vi "Fpga-ItchParser-TestHarness.vi"   [LabVIEW 2016]
uses:
  <vilib>/Platform/TimedLoop/XDataNode/timing_clust.ctl
  <vilib>/Platform/TimedLoop/XDataNode/nitl_modes.ctl
  <vilib>/Platform/TimedLoop/XDataNode/wakeup.ctl
  <vilib>/rvi/Emulation/niFpgaSctlEmulationGetInTimedLoop.vi
  <vilib>/rvi/Emulation/niFpgaEmulationReportErrorSimple.vi
  <vilib>/rvi/Emulation/niFpgaGetClockAttributes.vi
  <vilib>/rvi/Emulation/niFpgaCriticalErrorInLSC.vi
  <vilib>/rvi/interface/RandomDataEmulation/niFpgaRandomDataHandleErrors.vi
  <vilib>/rvi/Emulation/niFpgaEmulationIsFPGAContextNoSignature.vi
  <vilib>/rvi/errors/niFpgaSetErrorForExecOnDevCompSimple.vi
  <vilib>/rvi/eio/common/nirviEmuReportErrorAndStop.vi
  <vilib>/rvi/DataTransferAndStorage/Container/Common/niFpgaContainerGetUniqueNameForEmu.vi
  <vilib>/rvi/FIFO/Fifo_Resource/nirvififoEmulationSetSize.vi
  <vilib>/rvi/FIFO/Fifo_Resource/nirviFifoEmulationQueueMgr.vi
  <instcachedir>/0/nirviFifoEmulationQueueMgr_E5CAEC123FF24DC58D834DCA3CDAA9B5.lvgen/nirviFifoEmulationQueueMgr_E5CAEC123FF24DC58D834DCA3CDAA9B5_008.vi
  <vilib>/rvi/FIFO/Fifo_Resource/nirvififoEmulationDetermineInputValidOut.vi
  <vilib>/rvi/FIFO/Fifo_Resource/nirvififoEmulationCreateLock.vi
  <vilib>/rvi/Emulation/niFpgaProcessEmulError.vi
  <vilib>/rvi/FIFO/Fifo_Resource/nirvififoEmulationObtainLock.vi
  <vilib>/rvi/FIFO/Fifo_Resource/nirvififoEmulationReleaseLock.vi
  <vilib>/rvi/occurrence/nirviWaitOnOccurrenceBase.vi
  <vilib>/rvi/errors/nirviReportUnexpectedCaseInternalError.vi
  <vilib>/rvi/errors/nirviReportUnexpectedCaseInternalError (U32).vi
  <instcachedir>/0/nirviFifoEmulationQueueMgr_E5CAEC123FF24DC58D834DCA3CDAA9B5.lvgen/nirviFifoEmulationQueueMgr_E5CAEC123FF24DC58D834DCA3CDAA9B5_009.vi
  <vilib>/Utility/error.llb/Clear Errors.vi
  <vilib>/Platform/TimedLoop/XDataNode/XDataNode.xnode
  <vilib>/rvi/DataTransferAndStorage/Container/XNode/niFpgaContainer.xnode
  <vilib>/rvi/interface/RandomDataEmulation/nirviRandomDataFpgaReadWriteTemplate.vi
  <vilib>/rvi/FIFO/Fifo_Resource/nirvififoEmulationWrite.vi
  <vilib>/rvi/FIFO/Fifo_Resource/nirvififoEmulationRead.vi
  <vilib>/Platform/TimedLoop/XDataNode/XDNodeRunTimeDep.lvlib
types:
  T1 = cluster{"Operation":enum16{"Noop", "GetAll", "AddOrder", "DeleteOrder"}, "Cluster":cluster{"Side":u16, "OrderRefNum":u64, "Price":u32, "Shares":u32}}
  T2 = typedef "XDNodeRunTimeDep.lvlib/timing_clust.ctl" = cluster{"Expected End [f-1]":u64, "Actual End [f-1]":u64, "Finished Late? [f-1]":bool, "Expected End [i-1]":u64, "Actual End [i-1]":u64, "Finished Late? [i-1]":bool, "Expected Start [i]":u64, "Actual Start [i]":u64, "Expected Start [f]":u64, "Actual Start [f]":u64, "Source Name":string, "Structure Name":string, "Period":i64, "Deadline":i64, "Offset":i64, "Start":i64, "Priority":i32, "Timeout":i32, "Mode":T3, "Wakeup Reason":T4, "Error":errorcluster, "Source Type":string, "Secondary Source Type":string, "Global End Time":u64, "Global Start Time":u64, "Frame Duration":u64, "Iteration Duration":u64, "Assigned CPU":i32, "I/O Scan Engine Mode":u32}
  T3 = typedef "XDNodeRunTimeDep.lvlib/nitl_modes.ctl" = enum32{"No Change", "Process missed periods, maintain original phase", "Discard missed periods, maintain original phase", "Process missed periods, ignore original phase", "Discard missed periods, ignore original phase"}
  T4 = typedef "XDNodeRunTimeDep.lvlib/wakeup.ctl" = enum32{"Normal", "Aborted", "Asynchronous wakeup", "Timing source error", "Timed loop error", "Timeout"}
  T5 = enum16{"Noop", "GetAll", "AddOrder", "DeleteOrder"}
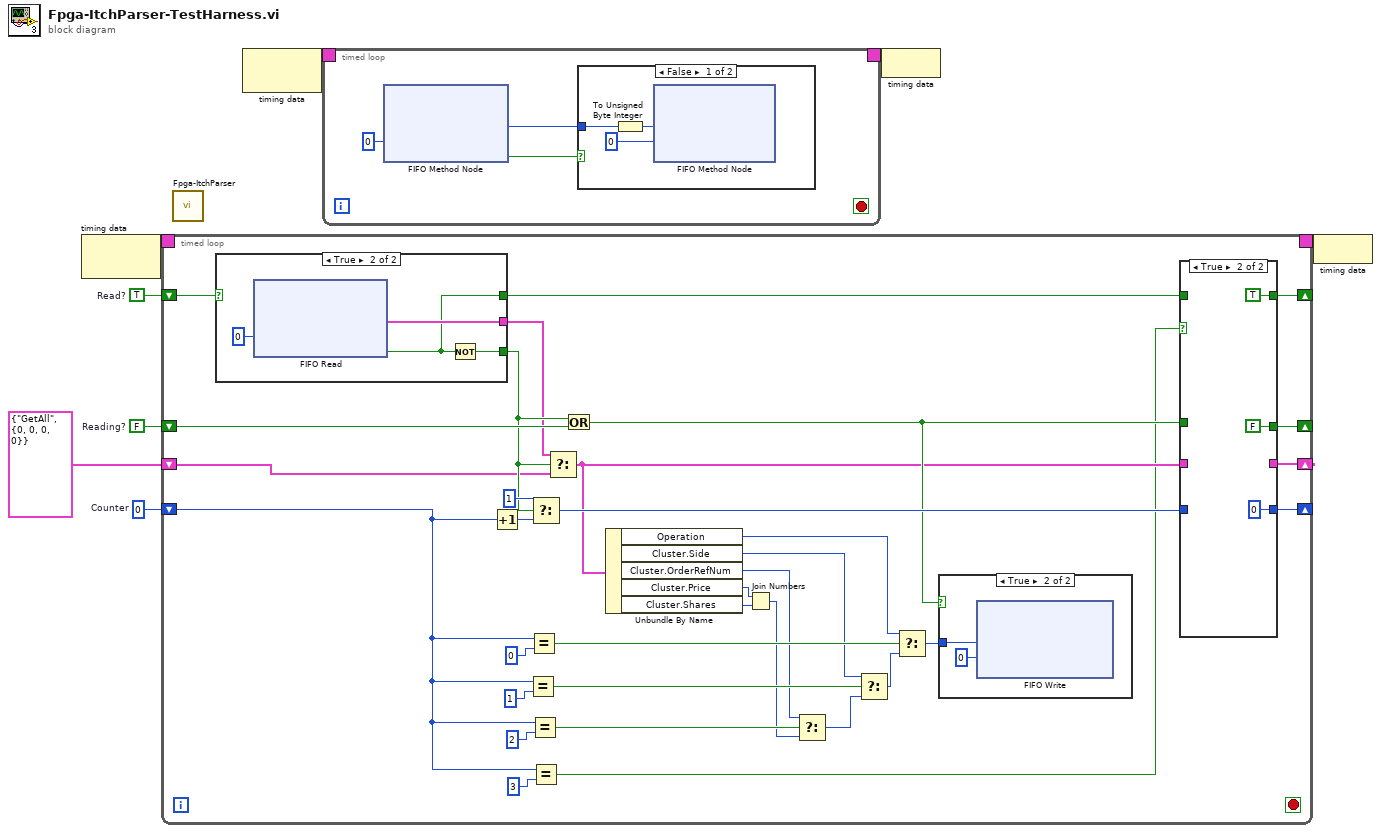
[diagram p0: block diagram]
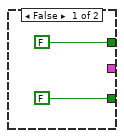
[diagram p4: hidden frame]
diagram:
  w2 = FALSE  # Reading?
  w3 = i16 0  # Counter
  w4 = TRUE  # Read?
  n1 = node-c288() -> (w6:T2)  [unwired: 1 in]
  n2 = timed-loop {
    timing: w6 -> [_]
    timing-out: [_] -> w5
    shift-right: [w39] -> _
    shift-left: w4 -> [w40]
    shift-right: [w37] -> _
    shift-left: w3 -> [w16]
    shift-right: [w35] -> _
    shift-left: w2 -> [w36]
    shift-right: [w29] -> _
    shift-left: T1 {"Operation"=enum."GetAll", "Cluster"={"Side"=0, "OrderRefNum"=0, "Price"=0, "Shares"=0}} ("OrderBookCommand") -> [w28]
    stop <- _ stop-if-true
    n3 = case shown="True" w40 {
      tunnel: [_ w55] -> w31
      tunnel: [FALSE ("Timed Out?") w54] -> w32
      tunnel: [FALSE w53] -> w38
      frame False {
      }
      frame True {
        n4 = xnode "FIFO Read"("Timeout"=0) -> ("Element"=w55:T1, "Timed Out?"=w53:bool)  [unwired: 1 in, 1 out]
        n5 = Not(x=w53) -> (.not. x?=w54:bool)
      }
    }
    n6 = Increment(x=w16) -> (x+1=w41:i16)
    n7 = Equal?(x=w16, y=i16 1) -> (x = y?=w22:bool)
    n8 = Equal?(x=w16, y=i16 0) -> (x = y?=w24:bool)
    n9 = Equal?(x=w16, y=i16 2) -> (x = y?=w13:bool)
    n10 = Select(t=i16 1, s=w32, f=w41) -> (s? t:f=w33:i16)
    n11 = Equal?(x=w16, y=i16 3) -> (x = y?=w14:bool)
    n12 = Select(t=w31, s=w32, f=w28) -> (s? t:f=w20:T1)
    n13 = Or(x=w32, y=w36) -> (x .or. y?=w30:bool)
    n14 = Unbundle By Name(w20) -> ("Operation"=w19:T5, "Cluster.Side"=w18:u16, "Cluster.OrderRefNum"=w12:u64, "Cluster.Price"=w11:u32, "Cluster.Shares"=w10:u32)
    n15 = Join Numbers(hi=w11, lo=w10) -> ((hi.lo)=w9:u64)
    n16 = Select(t=w12, s=w13, f=w9) -> (s? t:f=w15:u64)
    n17 = Select(t=w18, s=w22, f=w15) -> (s? t:f=w23:u64)
    n18 = Select(t=w19, s=w24, f=w23) -> (s? t:f=w21:u64)
    n19 = case shown="True" w30 {
      tunnel: w21 -> [_ w42]
      frame False {
      }
      frame True {
        n20 = xnode "FIFO Write"("Element"=w42, "Timeout"=0) -> ()  [unwired: 1 in, 2 out]
      }
    }
    n21 = case shown="True" w14 {
      tunnel: [w47 TRUE ("Timed Out?")] -> w39
      tunnel: w38 -> [w47 _]
      tunnel: w33 -> [w46 _]
      tunnel: [w46 i16 0 ("Counter")] -> w37
      tunnel: w30 -> [w45 _]
      tunnel: [w45 FALSE] -> w35
      tunnel: [w44 _] -> w29
      tunnel: w20 -> [w44 _]
      frame False {
      }
      frame True {
      }
    }
  }
  n22 = call "Fpga-ItchParser.vi"() -> ()  [unwired: 12 in]
  n23 = node-c288() -> (w8:T2)  [unwired: 1 in]
  n24 = timed-loop {
    timing: w8 -> [_]
    timing-out: [_] -> w7
    stop <- _ stop-if-true
    n25 = xnode ("FIFO Method Node")("Timeout"=0) -> ("Element"=w59:u8, "Timed Out?"=w60:bool)  [unwired: 1 in, 1 out]
    n26 = case shown="False" w60 {
      tunnel: w59 -> [w63 _]
      frame False {
        n27 = To Unsigned Byte Integer(number=w63) -> (unsigned 8bit integer=w62:u8)
        n28 = xnode ("FIFO Method Node")("Element"=w62, "Timeout"=0) -> ()  [unwired: 1 in, 2 out]
      }
      frame True {
      }
    }
  }
  n29 = node-c288(w7) -> ()
  n30 = node-c288(w5) -> ()
